vi "Pololu.Command Line Move Util.vi"(11 "Config Folder":path=path "C:/MTE/Camera_Calibration/Config") -> (0 "error out":errorcluster, 3 "Duration(s)":dbl)   [LabVIEW 2018]
uses:
  SubVIs/Pololu.Message Byte Defs.ctl
  Dual Servo Manager Class/PololuCtrl.lvclass
  <vilib>/KATE/Files/File Utils.lvlib
  <vilib>/KATE/Time/Time Utils.lvlib
panel:
  in  "Sim CL Args":string[](array[string])=["Move", "0"]
  out "CH 1 Pos":dbl
  out "CH 0 Pos":dbl
  in  "PID":string="0089"
  in  "VID":string="1FFB"
  in  "Test":bool
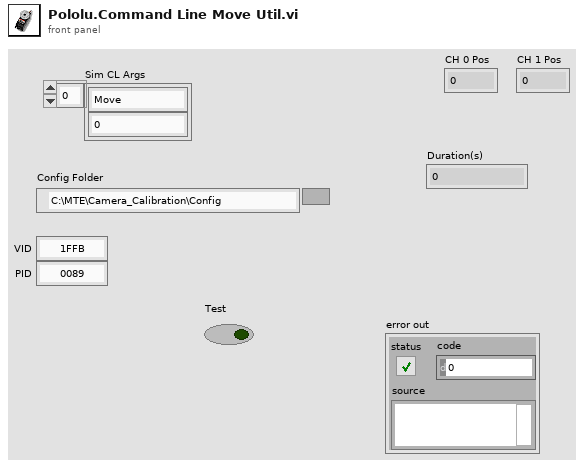
[diagram p1: front panel]
types:
  T1 = enum32{"Invalid", "Standard", "Closed", "Hidden", "Minimized", "Maximized"}
  T2 = enum32{"invalid app kind", "Development System", "Run Time System", "Student Edition", "Embedded LabVIEW", "Evaluation", "Custom"}
  T3 = typedef "Pololu.Message Byte Defs.ctl" = u8
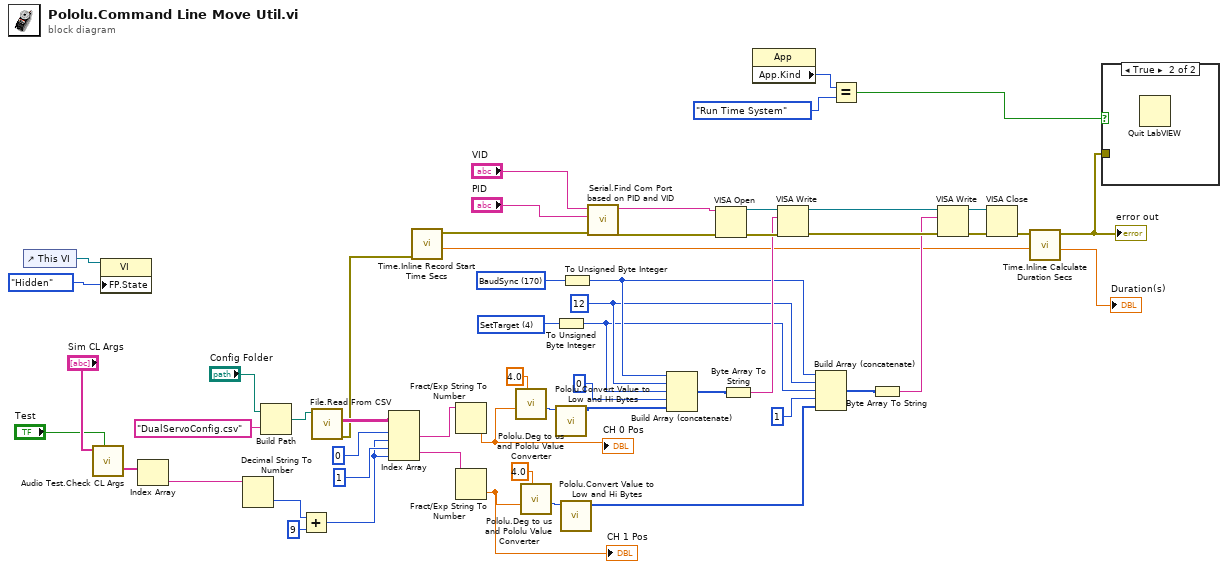
[diagram p0: block diagram]
diagram:
  w34 = 12
  w47 = T3 4 items=["BaudSync"=170, "SetTarget"=4, "Set Speed"=7, "Set Accel"=9, "Get Pos"=16, "Get MovStat"=19, "Get Errors"=33] ("Cmds")
  w48 = T3 170 items=["BaudSync"=170, "SetTarget"=4, "Set Speed"=7, "Set Accel"=9, "Get Pos"=16, "Get MovStat"=19, "Get Errors"=33] ("Cmds")
  n1 = control-ref of="This VI"() -> (w2:refnum<vi>)
  n2 = call "Audio Test.Check CL Args.vi"("Simulate"="Test", "Sim CL Args"="Sim CL Args") -> ("Args"=w26:string[])  [unwired: 7 in, 2 out]
  n3 = property class="VI"(reference=w2, "FP.State"=T1."Hidden" ("Front Panel Window:State")) -> ()  [unwired: 1 in, 2 out]
  n4 = Index Array(array=w26) -> (element=w22:string)  [unwired: 1 in]
  n5 = Decimal String To Number(string=w22) -> (number=w16:i32)  [unwired: 2 in, 1 out]
  n6 = Build Path(base path="Config Folder", name or relative path="DualServoConfig.csv") -> (appended path=w19:path)
  n7 = Add(x=w16, y=9 ("index (row)")) -> (x+y=w7:i32)
  n8 = call <vilib>:"File.Read From CSV.vi"("File"=w19) -> ("error out"=w9:errorcluster, "Data"=w25:string[][])  [unwired: 8 in, 1 out]
  n9 = Index Array(array=w25, index (row) #1=0 ("index (row)"), index (col) #1=w7, index (row) #2=1 ("index (row)"), index (col) #2=w7) -> (element #1=w21:string, element #2=w20:string)
  n10 = call <vilib>:"Time.Inline Record Start Time Secs.vi"("Error Out Lower"=w9) -> ("Start(s)"=w11:dbl, "Error Out Upper"=w12:errorcluster)  [unwired: 8 in, 1 out]
  n11 = Fract/Exp String To Number(string=w21) -> (number=w41:dbl)  [unwired: 3 in, 1 out]
  "CH 0 Pos" <- w41
  n12 = Fract/Exp String To Number(string=w20) -> (number=w8:dbl)  [unwired: 3 in, 1 out]
  "CH 1 Pos" <- w8
  n13 = call "Pololu.Deg to us and Pololu Value Converter.vi"("us to Units Mult"=4.0, "Set Pos (Deg)"=w41) -> ("Cmd units"=w42:u16)  [unwired: 8 in, 1 out]
  n14 = call "Pololu.Deg to us and Pololu Value Converter.vi"("us to Units Mult"=4.0, "Set Pos (Deg)"=w8) -> ("Cmd units"=w31:u16)  [unwired: 8 in, 1 out]
  n15 = To Unsigned Byte Integer(number=w47) -> (unsigned 8bit integer=w33:T3)
  n16 = call "Pololu.Convert Value to Low and Hi Bytes.vi"("Value"=w42) -> ("Low_Hi Bytes"=w49:u8[])  [unwired: 10 in]
  n17 = call "Pololu.Convert Value to Low and Hi Bytes.vi"("Value"=w31) -> ("Low_Hi Bytes"=w29:u8[])  [unwired: 10 in]
  n18 = To Unsigned Byte Integer(number=w48) -> (unsigned 8bit integer=w35:T3)
  n19 = call "Serial.Find Com Port based on PID and VID.vi"("error in"=w12, "PID"="PID", "VID"="VID") -> ("error out"=w50:errorcluster, "COM Port"=w51:string)  [unwired: 5 in, 2 out]
  n20 = Build Array (concatenate)(w35, w34, w33, 0, w49) -> (w45:i32[])
  n21 = VISA Open(error in (no error)=w50, VISA resource name=w51) -> (VISA resource name=w55:refnum<visa-resource-name>, error out=w54:errorcluster)  [unwired: 3 in]
  n22 = Byte Array To String(unsigned byte array=w45) -> (string=w44:string)
  n23 = property class="App"() -> ("App.Kind"=w5:T2)  [unwired: 2 in, 2 out]
  n24 = VISA Write(VISA resource name=w55, write buffer=w44, error in (no error)=w54) -> (VISA resource name out=w40:refnum<visa-resource-name>, error out=w39:errorcluster)  [unwired: 1 out]
  n25 = Build Array (concatenate)(w35, w34, w33, 1, w29) -> (w36:i32[])
  n26 = Equal?(x=w5, y=T2."Run Time System" ("Application:Kind")) -> (x = y?=w3:bool)
  n27 = Byte Array To String(unsigned byte array=w36) -> (string=w28:string)
  n28 = VISA Write(VISA resource name=w40, write buffer=w28, error in (no error)=w39) -> (VISA resource name out=w38:refnum<visa-resource-name>, error out=w37:errorcluster)  [unwired: 1 out]
  n29 = VISA Close(VISA resource name=w38, error in (no error)=w37) -> (error out=w13:errorcluster)
  n30 = call <vilib>:"Time.Inline Calculate Duration Secs.vi"("Start(Sec)"=w11, "Error In Top"=w13) -> ("Duration(s)"=→"Duration(s)":dbl, "Error Out Top"=w6:errorcluster)  [unwired: 7 in, 1 out]
  "error out" <- w6
  n31 = case shown="True" w3 {
    tunnel: w6 -> [_ _]
    frame False {
    }
    frame True {
      n32 = Quit LabVIEW() -> ()  [unwired: 1 in]
    }
  }
